vi "Function.vi"(8 "error in (no error)":errorcluster, 9 "Numeric B":u8, 10 "Numeric A":u8, 11 "Two Terminal in":refnum<class "Greater_U8.lvclass">) -> (0 "error out":errorcluster, 2 "Result":bool, 3 "Two Terminal out":refnum<class "Greater_U8.lvclass">)   [LabVIEW 2021, in "Greater_U8.lvclass"]
uses:
  Greater_U8.lvclass
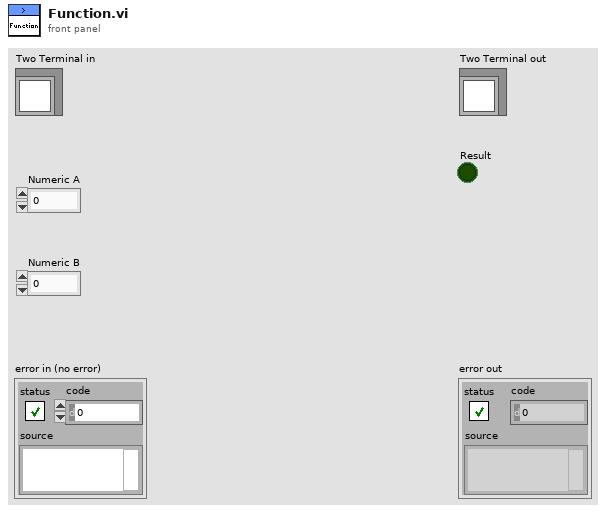
[diagram p1: front panel]
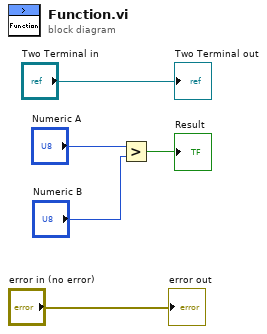
[diagram p0: block diagram]
diagram:
  n1 = Greater?(x="Numeric A", y="Numeric B") -> (0:→"Result":bool)
  "error out" <- "error in (no error)"
  "Two Terminal out" <- "Two Terminal in"
